vi "test3.vi"() -> ()   [LabVIEW 2018]
uses:
  <vilib>/imath/engines/lvmath/Plug In/_Char/NIMS_CH_character datatype.ctl
  <vilib>/imath/engines/lvmath2/RunTimeEngine/Managers/WorkSpace/UID Generator.vi
  <vilib>/imath/engines/lvmath/Plug In/_Char/NIMS_CH_Character RV to String.vi
  <vilib>/imath/engines/lvmath2/RunTimeEngine/BuiltInFunctions/random/NIMS_random.vi
  <vilib>/imathl/engines/lvmath/Functions/Error Handling/Create Error.vi
  <vilib>/imath/engines/lvmath2/RunTimeEngine/BuiltInFunctions/fir_win/NIMS_fir_win(I32,V,Str,V,Str).vi
  <vilib>/imath/engines/lvmath2/RunTimeEngine/ErrorHandling/NIMS_Create Error From Enums.vi
  <vilib>/imath/engines/lvmath2/RunTimeEngine/BuiltInFunctions/conv/NIMS_conv(M,M).vi
  <instcachedir>/0/NIMS_conv(M,M)_D972F9B3CDFC4C878A09791DEDB45279.lvgen/NIMS_conv(M,M)_D972F9B3CDFC4C878A09791DEDB45279_001.vi
  <vilib>/imath/engines/lvmath2/RunTimeEngine/ErrorHandling/NIMS_Error From Error Code.vi
  <vilib>/imath/engines/lvmath2/RunTimeSupport/NIMS_Get Any Vector_w Error - Matrix.vi
  <instcachedir>/0/NIMS_Get Any Vector_w Error - Matrix_1B26302039EC43C7B9FA287B1E12D88C.lvgen/NIMS_Get Any Vector_w Error - Matrix_1B26302039EC43C7B9FA287B1E12D88C_001.vi
  <vilib>/imath/engines/lvmath2/RunTimeEngine/BuiltInFunctions/psd_periodogram/NIMS_psd_periodogram().vi
  <instcachedir>/0/NIMS_psd_periodogram()_02030E41DB254B5B8F4838052F408B46.lvgen/NIMS_psd_periodogram()_02030E41DB254B5B8F4838052F408B46_000.vi
  <vilib>/imath/engines/lvmath2/RunTimeEngine/RunTimeType/NIMS_RunTimeType_From StrictType (excl LVString).vi
  <instcachedir>/0/NIMS_RunTimeType_From StrictType (excl LVString)_E7E34A65C99947108168652BAD14964D.lvgen/NIMS_RunTimeType_From StrictType (excl LVString)_E7E34A65C99947108168652BAD14964D_000.vi
  <vilib>/imath/engines/lvmath2/RunTimeEngine/LocalVariableDefStatement/MC_LocalVariableDefStatement_Display.vi
  <vilib>/imath/engines/lvmath2/RunTimeEngine/BuiltInFunctions/var/NIMS_var(GM,RV).vi
  <instcachedir>/0/NIMS_var(GM,RV)_40927390FCFA4ADD9C7A628E541F4120.lvgen/NIMS_var(GM,RV)_40927390FCFA4ADD9C7A628E541F4120_001.vi
  <vilib>/imath/engines/lvmath2/RunTimeEngine/ArithmeticOperatorToken/NIMS_ArithmeticOperator_rightdivmx(C,C).vi
  <instcachedir>/0/NIMS_ArithmeticOperator_rightdivmx(C,C)_3485B7D8BD804A089AB36E8AD92CB592.lvgen/NIMS_ArithmeticOperator_rightdivmx(C,C)_3485B7D8BD804A089AB36E8AD92CB592_000.vi
  <vilib>/imath/engines/lvmath2/RunTimeEngine/BuiltInFunctions/hilbert/NIMS_hilbert(RM, I32).vi
  <vilib>/imath/engines/lvmath2/RunTimeEngine/BuiltInFunctions/imag/NIMS_imag(Complex).vi
  <instcachedir>/0/NIMS_imag(Complex)_3180D40D00C843A49C2B33397F857BF3.lvgen/NIMS_imag(Complex)_3180D40D00C843A49C2B33397F857BF3_001.vi
  <vilib>/imath/engines/lvmath2/RunTimeEngine/BuiltInFunctions/size/NIMS_[I32,I32]=size(GM).vi
  <instcachedir>/0/NIMS_[I32,I32]=size(GM)_B0A6EC1255BB4C8AB801FE6F734128D9.lvgen/NIMS_[I32,I32]=size(GM)_B0A6EC1255BB4C8AB801FE6F734128D9_004.vi
  <vilib>/imath/engines/lvmath2/RunTimeEngine/RangeToken/NIMS_Range.vi
  <instcachedir>/0/NIMS_Range_846134F467D14A349F7C6CCEF459CDB2.lvgen/NIMS_Range_846134F467D14A349F7C6CCEF459CDB2_000.vi
  <vilib>/imath/engines/lvmath2/RunTimeEngine/ArithmeticOperatorToken/NIMS_ArithmeticOperator_times.vi
  <instcachedir>/0/NIMS_ArithmeticOperator_times_D7E4A7A4AD2C4409A0CE309D2741A5B4.lvgen/NIMS_ArithmeticOperator_times_D7E4A7A4AD2C4409A0CE309D2741A5B4_008.vi
  <instcachedir>/0/NIMS_ArithmeticOperator_times_D7E4A7A4AD2C4409A0CE309D2741A5B4.lvgen/NIMS_ArithmeticOperator_times_D7E4A7A4AD2C4409A0CE309D2741A5B4_007.vi
  <vilib>/imath/engines/lvmath2/RunTimeEngine/ArithmeticOperatorToken/NIMS_ArithmeticOperator_plus.vi
  <instcachedir>/0/NIMS_ArithmeticOperator_plus_DE670E32103C4C10ADF2A97367172B30.lvgen/NIMS_ArithmeticOperator_plus_DE670E32103C4C10ADF2A97367172B30_011.vi
  <vilib>/imath/engines/lvmath2/RunTimeEngine/ArithmeticOperatorToken/NIMS_ArithmeticOperator_minus.vi
  <instcachedir>/0/NIMS_ArithmeticOperator_minus_C4D0373119CC411691B2E50DF2E09F22.lvgen/NIMS_ArithmeticOperator_minus_C4D0373119CC411691B2E50DF2E09F22_009.vi
  <vilib>/imath/engines/lvmath2/RunTimeEngine/ArithmeticOperatorToken/NIMS_ArithmeticOperator_rightdiv(C,C).vi
  <instcachedir>/0/NIMS_ArithmeticOperator_rightdiv(C,C)_8E8B35E9E3BF47BFB716DE35A4F53DF6.lvgen/NIMS_ArithmeticOperator_rightdiv(C,C)_8E8B35E9E3BF47BFB716DE35A4F53DF6_001.vi
  <vilib>/imath/engines/lvmath2/RunTimeEngine/BuiltInFunctions/atan/NIMS_atan(C).vi
  <instcachedir>/0/NIMS_atan(C)_8B6477E860DC46CCB680487DA133A85D.lvgen/NIMS_atan(C)_8B6477E860DC46CCB680487DA133A85D_000.vi
  <instcachedir>/0/NIMS_ArithmeticOperator_times_D7E4A7A4AD2C4409A0CE309D2741A5B4.lvgen/NIMS_ArithmeticOperator_times_D7E4A7A4AD2C4409A0CE309D2741A5B4_001.vi
  <instcachedir>/0/NIMS_ArithmeticOperator_plus_DE670E32103C4C10ADF2A97367172B30.lvgen/NIMS_ArithmeticOperator_plus_DE670E32103C4C10ADF2A97367172B30_002.vi
  <vilib>/imath/engines/lvmath2/RunTimeSupport/NIMS_Complex To Real.vi
  <instcachedir>/0/NIMS_Complex To Real_DC07FF5F56D84FD694198341FF08C5E7.lvgen/NIMS_Complex To Real_DC07FF5F56D84FD694198341FF08C5E7_000.vi
  <vilib>/imath/engines/lvmath2/RunTimeEngine/BuiltInFunctions/histogram/NIMS_[M]=histogram(M).vi
  <vilib>/imath/engines/lvmath2/RunTimeEngine/Managers/SymbolTable/Clear UID.vi
  <vilib>/imath/engines/lvmath2/RunTimeEngine/NodeEndStatement/NIMS_NodeEndStatement_Output.vi
  <instcachedir>/0/NIMS_NodeEndStatement_Output_53EC0D466D134D7ABD903AC30B43404B.lvgen/NIMS_NodeEndStatement_Output_53EC0D466D134D7ABD903AC30B43404B_012.vi
  <instcachedir>/0/NIMS_NodeEndStatement_Output_53EC0D466D134D7ABD903AC30B43404B.lvgen/NIMS_NodeEndStatement_Output_53EC0D466D134D7ABD903AC30B43404B_003.vi
  <instcachedir>/0/NIMS_NodeEndStatement_Output_53EC0D466D134D7ABD903AC30B43404B.lvgen/NIMS_NodeEndStatement_Output_53EC0D466D134D7ABD903AC30B43404B_005.vi
  <vilib>/imath/engines/lvmath2/RunTimeEngine/ErrorHandling/NIMS_Finalize Error.vi
  <vilib>/imath/engines/lvmath2/RunTimeEngine/Managers/SymbolTable/NIMS_WorkSpace.lvlib
panel:
  out "X(t)":dbl[][](graph)
  out "包络平方值的分布直方图":i32[][](graph)
  out "包络A(t)样本值的分布直方图":i32[][](graph)
  out "相位样本值的分布直方图":i32[][](graph)
  out "包络平方值波形":dbl[][](graph)
  out "相位样本波形":dbl[][](graph)
  out "包络A(t)样本波形":dbl[][](graph)
  out "窄带信号功率谱密度":dbl[](graph)
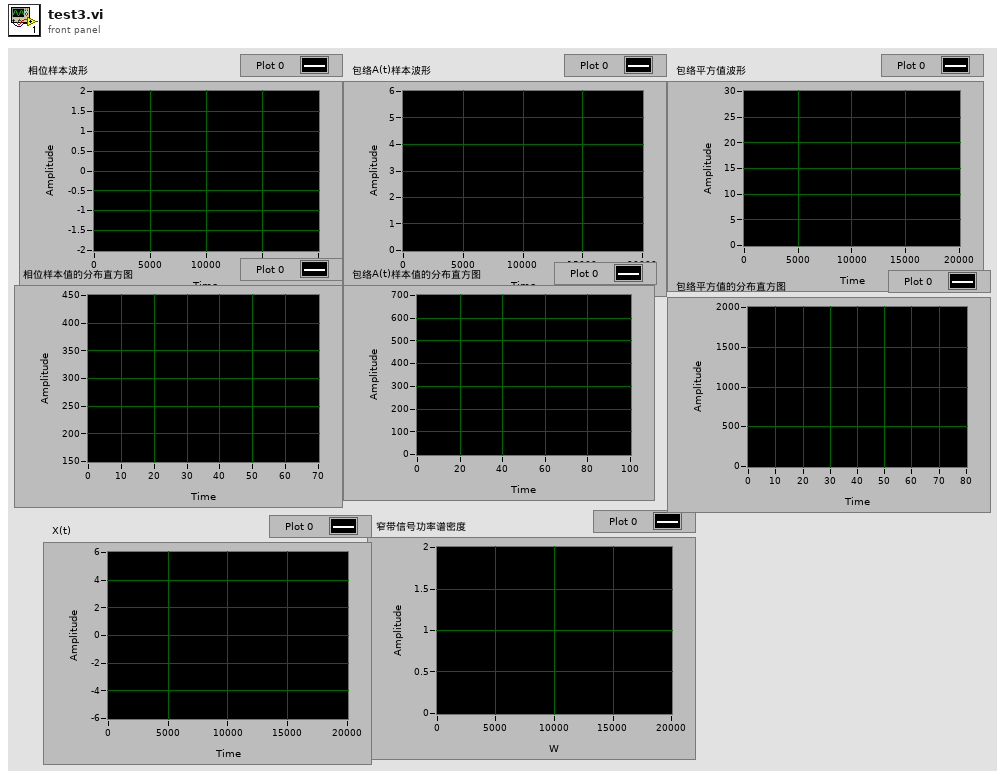
[diagram p1: front panel]
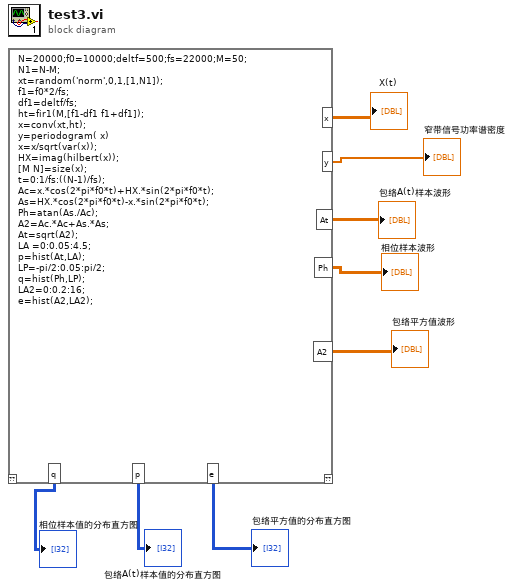
[diagram p0: block diagram]
diagram:
  n1 = mathscript code="N=20000;f0=10000;deltf=500;fs=22000;M=50;\nN1=N-M;\nxt=random('norm',0,1,[1,N1]);\nf1=f0*2/fs;\ndf1=deltf/fs;\nht=fir1(M,[f1-df1 f1+df1]);\nx=conv(xt,ht);\ny=periodogram( x)\nx=x/sqrt(var(x));                    \nHX=imag(hilbert(x));\n[M N]=size(x);\nt=0:1/fs:((N-1)/fs);\nAc=x.*cos(2*pi*f0*t)+HX.*sin(2*pi*f0*t);\nAs=HX.*cos(2*pi*f0*t)-x.*sin(2*pi*f0*t);\nPh=atan(As./Ac);\nA2=Ac.*Ac+As.*As;\nAt=sqrt(A2);\nLA =0:0.05:4.5;              \np=hist(At,LA);         \nLP=-pi/2:0.05:pi/2;                    \nq=hist(Ph,LP);             \nLA2=0:0.2:16;                      \ne=hist(A2,LA2);"() -> ("x"=→"X(t)":cdb[][], "y"=→"窄带信号功率谱密度":dbl[], "At"=→"包络A(t)样本波形":cdb[][], "Ph"=→"相位样本波形":cdb[][], "A2"=→"包络平方值波形":cdb[][], "q"=→"相位样本值的分布直方图":i32[][], "p"=→"包络A(t)样本值的分布直方图":i32[][], "e"=→"包络平方值的分布直方图":i32[][])  [unwired: 1 in, 1 out]
